vi "Write Pressure Servo Force Setpoint.vi"(10 "Pressure Servo Force Setpoint":dbl[unit], 11 "Model in":refnum<class "Model.lvclass">) -> (3 "Model out":refnum<class "Model.lvclass">)   [LabVIEW 2015, in "Model.lvclass"]
uses:
  Model.lvclass
  Model.lvclass/Model.ctl
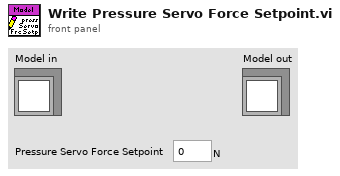
[diagram p1: front panel]
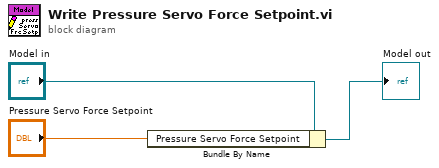
[diagram p0: block diagram]
diagram:
  n1 = Bundle By Name(cluster="Model in", "Pressure Servo Force Setpoint"="Pressure Servo Force Setpoint") -> (→"Model out":refnum<class "Model.lvclass">)
